vi "Execute OpenTypeDef-RunTime.vi"(6 "Mouse Position":T1, 8 "User VI Ref":refnum<vi>, 9 "Menu Item Tag Suffix":string, 10 "Remaining Items":refnum<vi>[](array[refnum]), 11 "Affected Items":T2) -> (0 "Fail transaction?":bool)   [LabVIEW 2020]
doc: "This VI is part of a plug-in for modifying the LabVIEW shortcut menus. This is the execute VI which is called when the shortcut menu is chosen by the user. It performs the action of the selected menu item."
uses:
  OpenTypeDef-RunTime.ctl
  <vilib>/Utility/miscctls.llb/LVPositionTypeDef.ctl
panel:
  # "All controls on this panel except \"Affected Items\" have been locked to prevent accidental edits. Changing the control names or types, other than the elements of the \"Affected Items\" cluster will make the VI unusable as a menu plugin.\n\nSee Context Help for each control for details about its use."
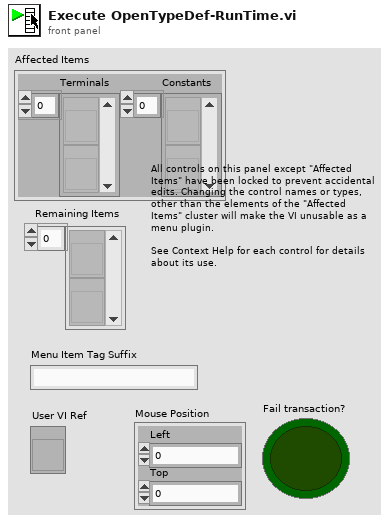
[diagram p1: front panel]
types:
  T1 = typedef "LVPositionTypeDef.ctl" = cluster{"Left":i32, "Top":i32}
  T2 = typedef "OpenTypeDef-RunTime.ctl" = cluster{"Terminals":refnum<vi>[], "Constants":refnum<vi>[]}
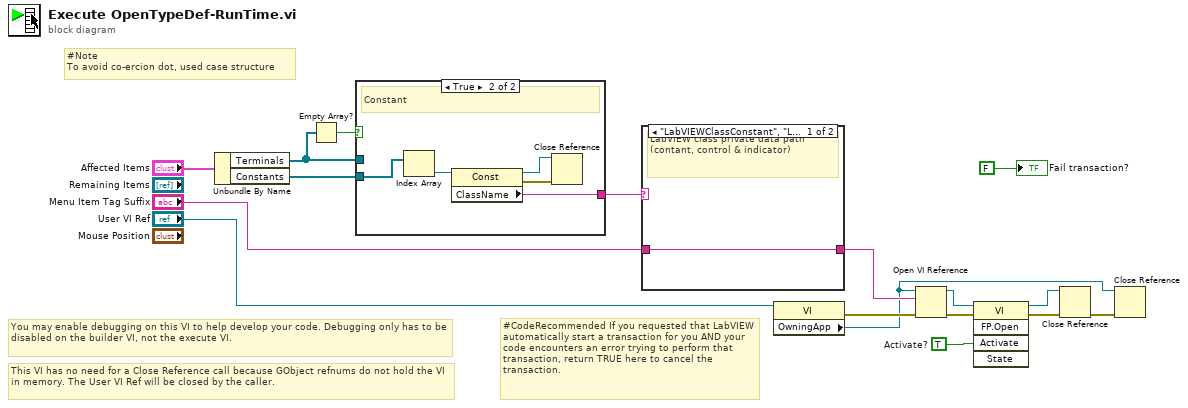
[diagram p0: block diagram]
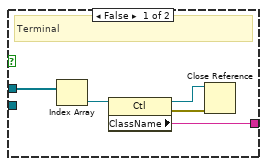
[diagram p2: hidden frame]
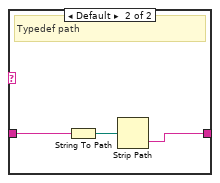
[diagram p3: hidden frame]
diagram:
  w11 = TRUE  # Activate?
  # "#Note\nTo avoid co-ercion dot, used case structure"
  # "You may enable debugging on this VI to help develop your code. Debugging only has to be disabled on the builder VI, not the execute VI."
  # "#CodeRecommended If you requested that LabVIEW automatically start a transaction for you AND your code encounters an error trying to perform that transaction, return TRUE here to cancel the transaction."
  # "This VI has no need for a Close Reference call because GObject refnums do not hold the VI in memory. The User VI Ref will be closed by the caller."
  n1 = Unbundle By Name("Affected Items") -> ("Terminals"=w3:refnum<vi>[], "Constants"=w2:refnum<vi>[])
  n2 = Empty Array?(array=w3) -> (empty?=w4:bool)
  n3 = case shown="True" w4 {
    tunnel: w3 -> [w21 _]
    tunnel: w2 -> [_ w23]
    tunnel: [w20 w26] -> w1
    frame False {
      # "Terminal"
      n4 = Index Array(array=w21) -> (element=w22:refnum<vi>)  [unwired: 1 in]
      n5 = property class="Ctl"(reference=w22) -> (reference out=w18:refnum<vi>, error out=w19:errorcluster, "ClassName"=w20:string)  [unwired: 1 in]
      n6 = Close Reference(reference=w18, error in (no error)=w19) -> ()  [unwired: 1 out]
    }
    frame True {
      # "Constant"
      n7 = Index Array(array=w23) -> (element=w27:refnum<vi>)  [unwired: 1 in]
      n8 = property class="Const"(reference=w27) -> (reference out=w24:refnum<vi>, error out=w25:errorcluster, "ClassName"=w26:string)  [unwired: 1 in]
      n9 = Close Reference(reference=w24, error in (no error)=w25) -> ()  [unwired: 1 out]
    }
  }
  n10 = case shown="\"LabVIEWClassConstant\", \"LabVIEWClassControl\"" w1 {
    tunnel: "Menu Item Tag Suffix" -> [w28 w30]
    tunnel: [w28 w29] -> w17
    frame "LabVIEWClassConstant", "LabVIEWClassControl" {
      # "LabVIEW class private data path (contant, control & indicator)"
    }
    frame Default {
      # "Typedef path"
      n11 = String To Path(string=w30) -> (path=w31:path)
      n12 = Strip Path(path=w31) -> (name=w29:string)  [unwired: 1 out]
    }
  }
  n13 = property class="VI"(reference="User VI Ref") -> (error out=w14:errorcluster, "OwningApp"=w6:refnum<vi>)  [unwired: 1 in, 1 out]
  n14 = Open VI Reference(application reference (local)=w6, vi path=w17, error in (no error)=w14) -> (vi reference=w7:refnum<vi>, error out=w12:errorcluster)  [unwired: 3 in]
  n15 = invoke class="VI" method="FP.Open"(reference=w7, error in=w12, "Activate"=w11) -> (reference out=w9:refnum<vi>, error out=w10:errorcluster)  [unwired: 2 in, 3 out]
  n16 = Close Reference(reference=w9, error in (no error)=w10) -> (error out=w8:errorcluster)
  n17 = Close Reference(reference=w6, error in (no error)=w8) -> ()  [unwired: 1 out]
  "Fail transaction?" <- FALSE ("Fail transaction?")
